vi "testRSAEncrypt&Decrypt.vi"(8 "error in (no error)":errorcluster, 11 "TestCase in":refnum<class "TestRSA.lvclass">) -> (0 "error out":errorcluster, 3 "TestCase out":refnum<class "TestRSA.lvclass">)   [LabVIEW 2021, in "TestRSA.lvclass"]
uses:
  TestRSA.lvclass
  Asymmetric Encryption/RSA/RSAEncryptionPadding.ctl
  <vilib>/addons/_JKI Toolkits/VI Tester/TestCase.llb/TestCase.lvclass
  Asymmetric Encryption/dotNET Crypto Asymmetric Encryption.lvlib
  Key Management/dotNET Crypto Key Management.lvlib
  C:/Program Files (x86)/National Instruments/LabVIEW 2021/vi.lib/addons/_JKI Toolkits/VI Tester/TestCase.llb/TestCase.lvclass
panel:
  out "Decrypted data":string
  out "Encrypted data":string
  out "Encrypted data out":u8[](array[numeric])
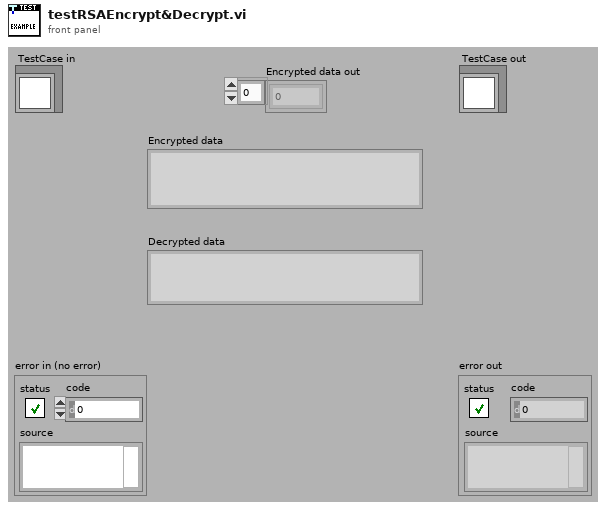
[diagram p1: front panel]
types:
  T1 = typedef "dotNET Crypto Asymmetric Encryption.lvlib/RSAEncryptionPadding.ctl" = enum16{"OaepSHA1", "OaepSHA256", "OaepSHA384", "OaepSHA512", "Pkcs1"}
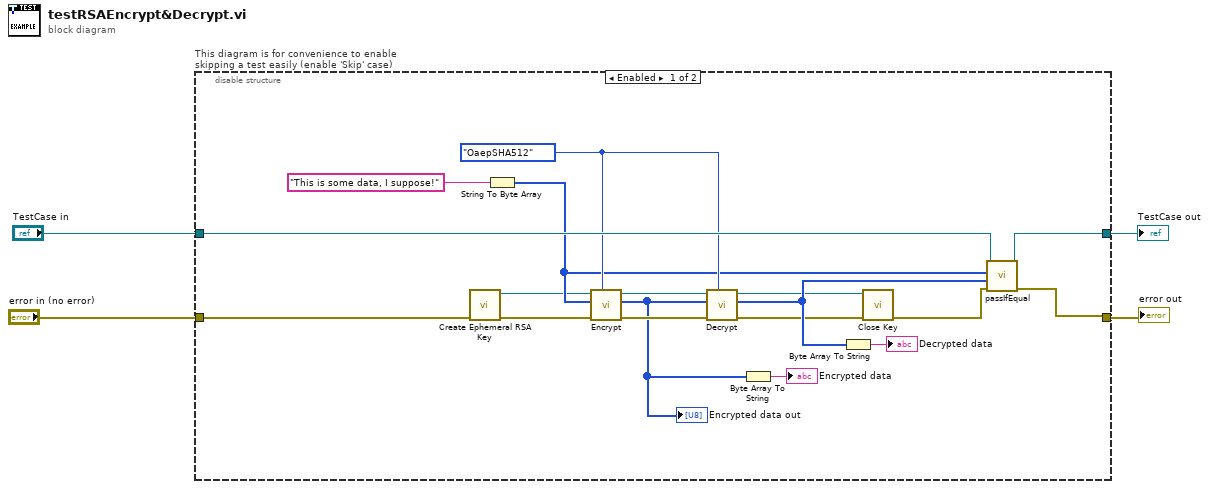
[diagram p0: block diagram]
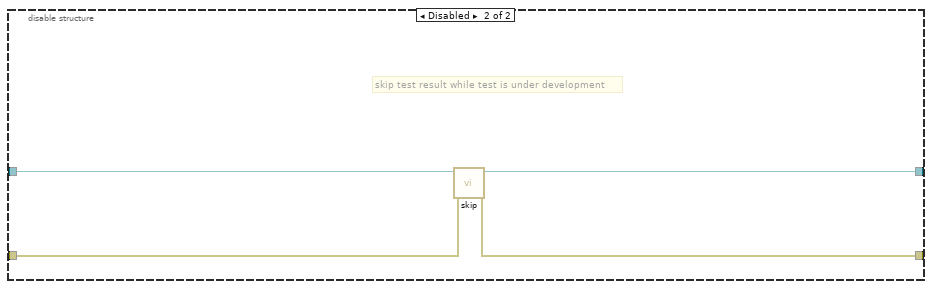
[diagram p2: hidden frame]
diagram:
  n1 = disable-structure "This diagram is for convenience to enable skipping a test easily (enable 'Skip' case)" shown="Enabled" {
    disable-tunnel: "TestCase in" -> [w22 w26]
    disable-tunnel: [w21 w24] -> w1
    disable-tunnel: [w20 w25] -> w3
    disable-tunnel: "error in (no error)" -> [w7 w23]
    frame Enabled {
      w18 = RSAEncryptionPadding."OaepSHA512" ("Padding Mode")
      n2 = call "Create Ephemeral RSA Key.vi"("error in (no error)"=w7) -> ("error out"=w6:errorcluster, "CngKey out"=w5:refnum<k24>)  [unwired: 9 in]
      n3 = String To Byte Array(string="This is some data, I suppose!") -> (unsigned byte array=w14:u8[])
      n4 = call "Encrypt.vi"("Padding Mode"=w18, "error in (no error)"=w6, "Raw data in"=w14, "CngKey in"=w5) -> ("error out"=w19:errorcluster, "Encrypted data out"=w12:u8[], "CngKey out"=w13:refnum<k24>)  [unwired: 5 in]
      "Encrypted data out" <- w12
      n5 = call "Decrypt.vi"("Padding Mode"=w18, "error in (no error)"=w19, "Encrypted data in"=w12, "CngKey in"=w13) -> ("error out"=w10:errorcluster, "Raw data out"=w11:u8[], "CngKey out"=w8:refnum<k24>)  [unwired: 5 in]
      n6 = Byte Array To String(unsigned byte array=w12) -> (string=→"Encrypted data":string)
      n7 = Byte Array To String(unsigned byte array=w11) -> (string=→"Decrypted data":string)
      n8 = call "Close Key.vi"("error in (no error)"=w10, "CngKey in"=w8) -> ("error out"=w9:errorcluster)  [unwired: 9 in]
      n9 = call-dynamic "passIfEqual.vi"("error in (no error)"=w9, "y"=w11, "x"=w14, "TestCase in"=w22) -> ("error out"=w20:errorcluster, "TestCase out"=w21:refnum<class "TestRSA.lvclass">)  [unwired: 6 in]
    }
    frame Disabled {
      # "skip test result while test is under development"
      n10 = call <vilib>:"skip.vi"("error in (no error)"=w23, "TestCase in"=w26) -> ("error out"=w25:errorcluster, "TestCase out"=w24:refnum<class "TestRSA.lvclass">)  [unwired: 8 in]
    }
  }
  "error out" <- w3
  "TestCase out" <- w1
